vi "Read client handle.vi"(8 "error in (no error)":errorcluster, 11 "OAuthClient in":refnum<class "OAuthClient.lvclass">) -> (0 "error out":errorcluster, 2 "Client Handle":T1, 3 "OAuthClient out":refnum<class "OAuthClient.lvclass">)   [LabVIEW 2013, in "OAuthClient.lvclass"]
uses:
  OAuthClient.lvclass
  <vilib>/httpClient/ClientHandle.ctl
  OAuthClient.lvclass/OAuthClient.ctl
  <vilib>/httpClient/LabVIEWHTTPClient.lvlib
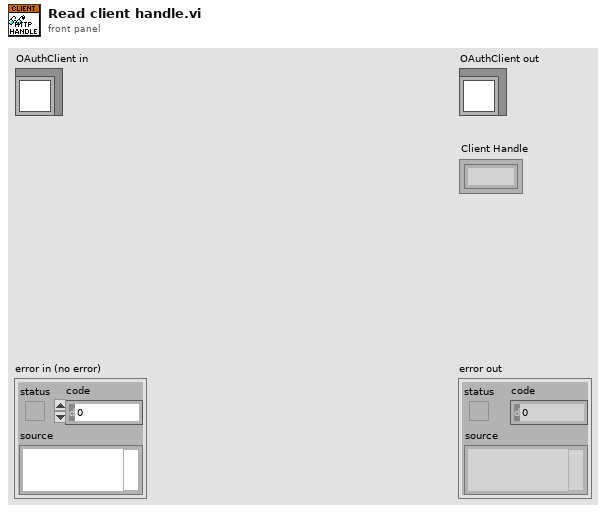
[diagram p1: front panel]
types:
  T1 = typedef "LabVIEWHTTPClient.lvlib/ClientHandle.ctl" = refnum<k1>
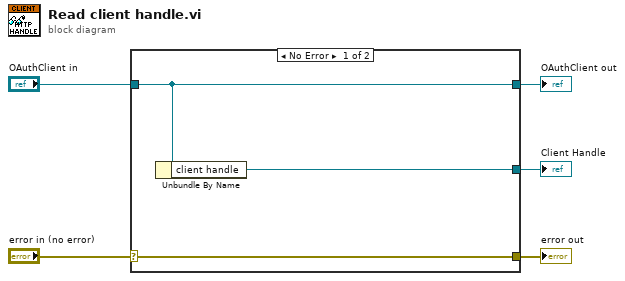
[diagram p0: block diagram]
diagram:
  n1 = case shown="No Error" "error in (no error)" {
    selector: "error in (no error)" -> [w8 w9]
    tunnel: [w8 w9] -> w4
    tunnel: [w7 w10] -> w2
    tunnel: "OAuthClient in" -> [w7 w10]
    tunnel: [w6 _] -> w1
    frame No Error {
      n2 = Unbundle By Name(w7) -> ("client handle"=w6:T1)
    }
    frame Error {
    }
  }
  "error out" <- w4
  "OAuthClient out" <- w2
  "Client Handle" <- w1
